vi "createPubDataEvents.vi"(8 "error in (no error)":errorcluster, 11 "UserEvents in":refnum<class "UserEvents.lvclass">) -> (0 "error out":errorcluster, 3 "UserEvents out":refnum<class "UserEvents.lvclass">)   [LabVIEW 2013, in "UserEvents.lvclass"]
uses:
  UserEvents.lvclass
  Typedefs/StateSelector.ctl
  Typedefs/OutputData.ctl
  UserEvents.lvclass/UserEvents.ctl
  Typedefs/ILCBTTypedefs.lvlib
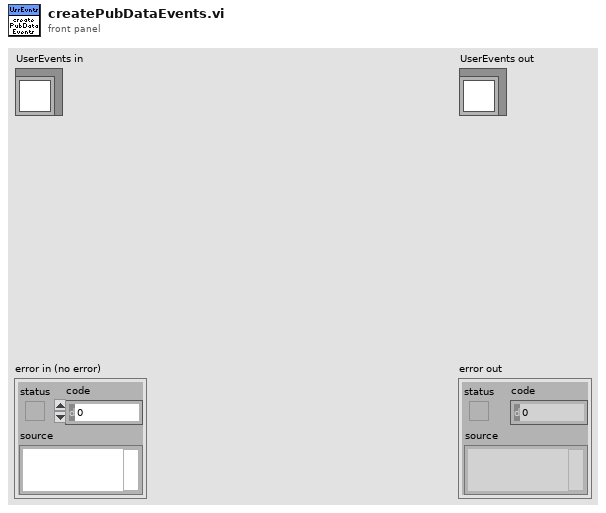
[diagram p1: front panel]
types:
  T1 = typedef "ILCBTTypedefs.lvlib/OutputData.ctl" = cluster{"Ch1":u16, "Ch2":u16, "Ch3":u16}
  T2 = typedef "ILCBTTypedefs.lvlib/StateSelector.ctl" = enum16{"EnabledState", "FaultState", "OffState", "StandbyState"}
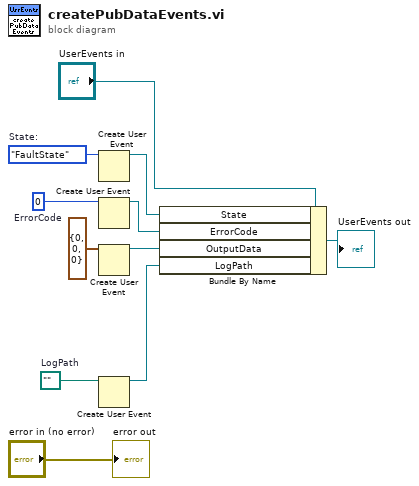
[diagram p0: block diagram]
diagram:
  w2 = path ""  # LogPath
  w7 = 0  # ErrorCode
  w8 = StateSelector."FaultState"  # State:
  n1 = Create User Event(user event datatype=w8) -> (user event=w6:refnum<user-event>)  [unwired: 1 in, 1 out]
  n2 = Create User Event(user event datatype=w7) -> (user event=w5:refnum<user-event>)  [unwired: 1 in, 1 out]
  n3 = Create User Event(user event datatype=T1 {"Ch1"=0, "Ch2"=0, "Ch3"=0} ("Output Data")) -> (user event=w3:refnum<user-event>)  [unwired: 1 in, 1 out]
  n4 = Create User Event(user event datatype=w2) -> (user event=w1:refnum<user-event>)  [unwired: 1 in, 1 out]
  n5 = Bundle By Name(cluster="UserEvents in", "State"=w6, "ErrorCode"=w5, "OutputData"=w3, "LogPath"=w1) -> (→"UserEvents out":refnum<class "UserEvents.lvclass">)
  "error out" <- "error in (no error)"
